vi "Get FPGA from Metadata.vi"(8 "error in (no error)":errorcluster, 10 "Device Model Str":string="myRIO", 11 "Title":string) -> (0 "error out":errorcluster, 1 "Customized?":bool, 2 "Supported FPGA Personalities":string[](array[string]), 3 "Defaul FPGA Personality":string, 4 "Found?":bool)   [LabVIEW 2021, in "Personality.lvlib"]
doc: "Gets the FPGA personality information from the myRIO project meta file with specified project title."
uses:
  <vilib>/myRIO/Common/FPGA Personality Framework/Personality.lvlib
  <vilib>/xml/Load XML File.vi
  <vilib>/xml/Close Reference(Node).vi
  <vilib>/xml/NI_XML.lvlib
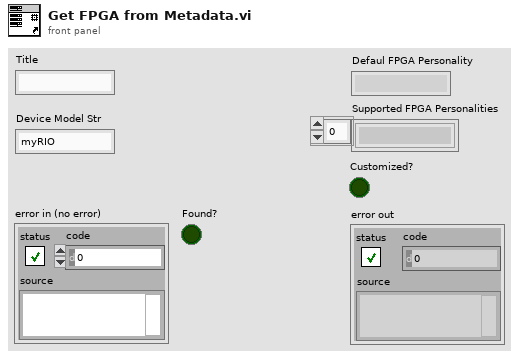
[diagram p1: front panel]
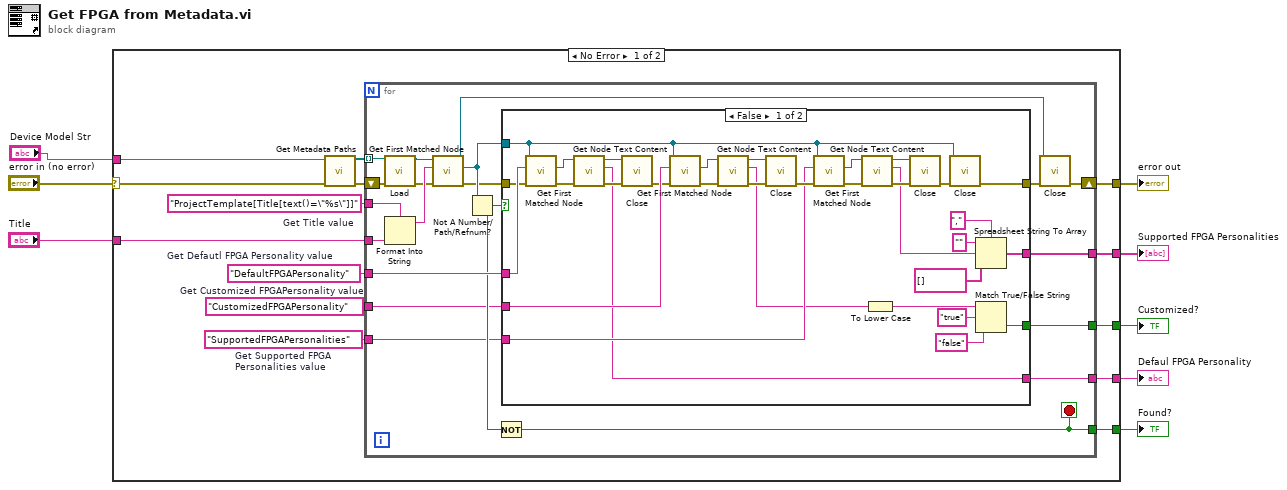
[diagram p0: block diagram]
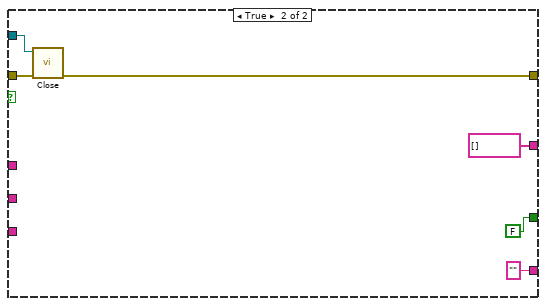
[diagram p2: hidden frame]
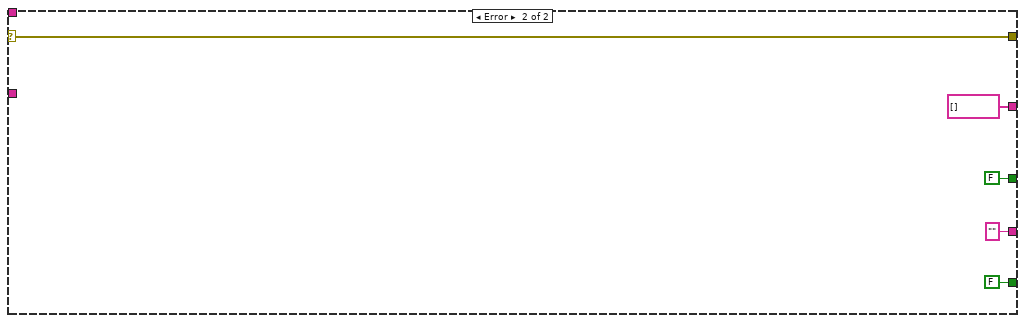
[diagram p3: hidden frame]
diagram:
  n1 = case shown="No Error" "error in (no error)" {
    selector: "error in (no error)" -> [w18 w85]
    tunnel: "Title" -> [w22 _]
    tunnel: [w21 "" ("node text")] -> w7
    tunnel: [w20 string[] [] ("Supported Fixed Personalities")] -> w6
    tunnel: [w19 w85] -> w5
    tunnel: [w11 FALSE ("selection")] -> w3
    tunnel: [w10 FALSE] -> w2
    tunnel: "Device Model Str" -> [w9 _]
    frame No Error {
      w13 = "CustomizedFPGAPersonality"  # Get Customized FPGAPersonality value
      w12 = "SupportedFPGAPersonalities"  # Get Supported FPGA Personalities value
      w16 = "DefaultFPGAPersonality"  # Get Defautl FPGA Personality value
      w17 = "ProjectTemplate[Title[text()=\"%s\"]]"  # Get Title value
      n2 = call <vilib>:"Get Metadata Paths.vi"("error in (no error)"=w18, "Device Model Str"=w9) -> ("error out"=w15:errorcluster, "Meta Data File Paths"=w14:path[])  [unwired: 8 in]
      n3 = for {
        tunnel: w22 -> [w42]
        tunnel: [w40] -> w21
        tunnel: [w39] -> w20
        tunnel: w17 -> [w37]
        tunnel: w16 -> [w35]
        tunnel: w14 -> [w28] mode=indexing
        shift-right: [w38] -> w19
        shift-left: w15 -> [w41]
        tunnel: w13 -> [w26]
        tunnel: w12 -> [w25]
        tunnel: [w24] -> w11
        tunnel: [w23] -> w10
        stop <- w23 stop-if-true
        n4 = call-poly <vilib>:"Load.vi"("path to XML document"=w28, "error in (no error)"=w41) -> ("DOM document out"=w34:refnum<k20>, "error out"=w33:errorcluster)  [unwired: 11 in, 1 out]
        n5 = Format Into String(format string=w37, w42) -> (resulting string=w36:string)  [unwired: 2 in, 1 out]
        n6 = call <vilib>:"Get First Matched Node.vi"("error in (no error)"=w33, "XPath expression"=w36, "node in"=w34) -> ("error out"=w30:errorcluster, "node result"=w32:refnum<k20>, "node out"=w29:refnum<k20>)  [unwired: 6 in]
        n7 = Not A Number/Path/Refnum?(number/path/refnum=w32) -> (NaN/Path/Refnum?=w27:bool)
        n8 = Not(x=w27) -> (.not. x?=w23:bool)
        n9 = case shown="False" w27 {
          tunnel: w35 -> [w74 _]
          tunnel: w32 -> [w50 w77]
          tunnel: [w48 "" ("node text")] -> w40
          tunnel: [w72 w78] -> w31
          tunnel: [w70 string[] [] ("Supported Fixed Personalities")] -> w39
          tunnel: w30 -> [w69 w79]
          tunnel: w26 -> [w54 _]
          tunnel: w25 -> [w51 _]
          tunnel: [w43 FALSE ("selection")] -> w24
          frame False {
            n10 = call <vilib>:"Get First Matched Node.vi"("error in (no error)"=w69, "XPath expression"=w74, "node in"=w50) -> ("error out"=w67:errorcluster, "node result"=w65:refnum<k20>)  [unwired: 6 in, 1 out]
            n11 = call <vilib>:"Get Node Text Content.vi"("error in (no error)"=w67, "node in"=w65) -> ("error out"=w66:errorcluster, "node text"=w48:string, "node out"=w64:refnum<k20>)  [unwired: 7 in]
            n12 = call-poly <vilib>:"Close.vi"("error in (no error)"=w66, "node"=w64) -> ("error out"=w53:errorcluster)  [unwired: 7 in]
            n13 = call <vilib>:"Get First Matched Node.vi"("error in (no error)"=w53, "XPath expression"=w54, "node in"=w50) -> ("error out"=w59:errorcluster, "node result"=w57:refnum<k20>)  [unwired: 6 in, 1 out]
            n14 = call <vilib>:"Get Node Text Content.vi"("error in (no error)"=w59, "node in"=w57) -> ("error out"=w58:errorcluster, "node text"=w47:string, "node out"=w56:refnum<k20>)  [unwired: 7 in]
            n15 = call-poly <vilib>:"Close.vi"("error in (no error)"=w58, "node"=w56) -> ("error out"=w52:errorcluster)  [unwired: 7 in]
            n16 = call <vilib>:"Get First Matched Node.vi"("error in (no error)"=w52, "XPath expression"=w51, "node in"=w50) -> ("error out"=w60:errorcluster, "node result"=w62:refnum<k20>)  [unwired: 6 in, 1 out]
            n17 = call <vilib>:"Get Node Text Content.vi"("error in (no error)"=w60, "node in"=w62) -> ("error out"=w61:errorcluster, "node text"=w49:string, "node out"=w63:refnum<k20>)  [unwired: 7 in]
            n18 = To Lower Case(string=w47) -> (all lower case string=w44:string)
            n19 = call-poly <vilib>:"Close.vi"("error in (no error)"=w61, "node"=w63) -> ("error out"=w55:errorcluster)  [unwired: 7 in]
            n20 = call-poly <vilib>:"Close.vi"("error in (no error)"=w55, "node"=w50) -> ("error out"=w72:errorcluster)  [unwired: 7 in]
            n21 = Spreadsheet String To Array(delimiter (Tab)=",", format string="", spreadsheet string=w49, array type (2D Dbl)=string[] [] ("Supported Fixed Personalities")) -> (array=w70:string[])
            n22 = Match True/False String(2:"false" ("false string"), 3:"true" ("true string"), 4:w44) -> (0:w43:bool)  [unwired: 1 out]
          }
          frame True {
            n23 = call-poly <vilib>:"Close.vi"("error in (no error)"=w79, "node"=w77) -> ("error out"=w78:errorcluster)  [unwired: 7 in]
          }
        }
        n24 = call-poly <vilib>:"Close.vi"("error in (no error)"=w31, "node"=w29) -> ("error out"=w38:errorcluster)  [unwired: 7 in]
      }
    }
    frame Error {
    }
  }
  "Defaul FPGA Personality" <- w7
  "Supported FPGA Personalities" <- w6
  "error out" <- w5
  "Customized?" <- w3
  "Found?" <- w2
